vi "Acquire SFTP.vi"(8 "error in (no error)":errorcluster, 11 "sftp":T1) -> (0 "error out":errorcluster, 2 "LIBSSH2_SFTP*":u64)   [LabVIEW 2017, in "libssh2.lvlib"]
uses:
  libssh2.lvlib
  SFTP Refnum.ctl
  <vilib>/Utility/semaphor.llb/Acquire Semaphore.vi
  Read Session Refnum.vi
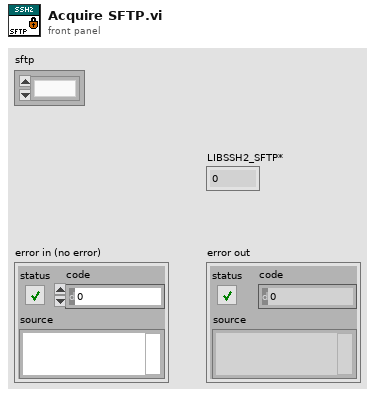
[diagram p1: front panel]
types:
  T1 = typedef "libssh2.lvlib/SFTP Refnum.ctl" = refnum<k1>
  T2 = typedef "libssh2.lvlib/Session Refnum.ctl" = refnum<k1>
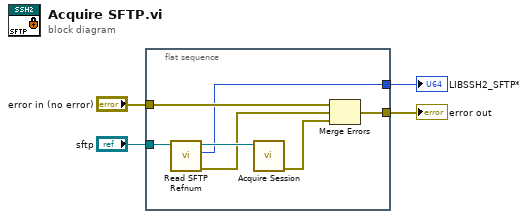
[diagram p0: block diagram]
diagram:
  n1 = flat-sequence {
    tunnel: [w8] -> w4
    tunnel: "error in (no error)" -> [w7]
    tunnel: "sftp" -> [w6]
    tunnel: [w5] -> w1
    frame #0 {
      n2 = call "Read SFTP Refnum.vi"("sftp"=w6) -> ("error out"=w10:errorcluster, "LIBSSH2_SFTP*"=w5:u64, "session"=w11:T2)  [unwired: 8 in]
      n3 = call "Acquire Session.vi"("session"=w11) -> ("error out"=w9:errorcluster)  [unwired: 8 in, 2 out]
      n4 = Merge Errors(w7, w10, w9) -> (w8:errorcluster)
    }
  }
  "error out" <- w4
  "LIBSSH2_SFTP*" <- w1
